vi "fg_authorization.vi"(8 "error in (no error)":errorcluster, 11 "authorization in":T1) -> (0 "error out":errorcluster, 3 "authorization out":T1)   [LabVIEW 2015, in "lv-dropbox.lvlib"]
uses:
  lv-dropbox.lvlib
  _controls/authorization.ctl
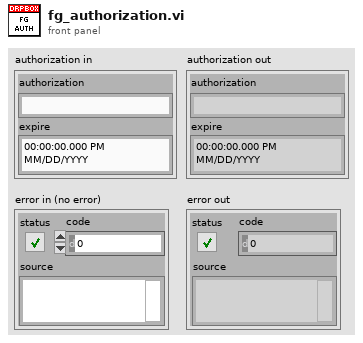
[diagram p1: front panel]
types:
  T1 = typedef "lv-dropbox.lvlib/authorization.ctl" = cluster{"authorization":string, "expire":timestamp}
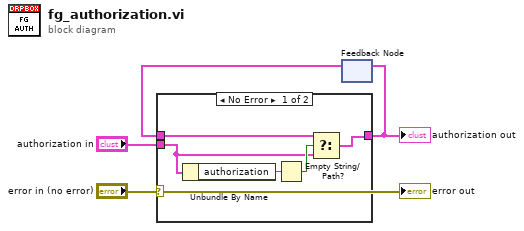
[diagram p0: block diagram]
diagram:
  n1 = feedback #1() -> (w3:T1)  [unwired: 1 in]
  n2 = case shown="No Error" "error in (no error)" {
    tunnel: [w9 w10] -> w4
    tunnel: w3 -> [w7 w10]
    tunnel: "authorization in" -> [w6 _]
    frame No Error {
      n3 = Unbundle By Name(w6) -> ("authorization"=w5:string)
      n4 = Empty String/Path?(string/path=w5) -> (empty?=w8:bool)
      n5 = Select(t=w7, s=w8, f=w6) -> (s? t:f=w9:T1)
    }
    frame Error {
    }
  }
  "authorization out" <- w4
  n6 = feedback-in #1(w4) -> ()
  "error out" <- "error in (no error)"
